vi "Die_Roller.vi"() -> ()   [LabVIEW 2020]
panel:
  out "FACE OCCURRENCES":T1
  out "Throws":dbl[](array[numeric])
  in  "Numeri Lanci":i32
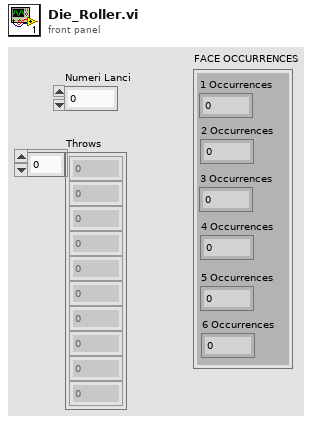
[diagram p1: front panel]
types:
  T1 = cluster{"1 Occurrences":dbl, "2 Occurrences":dbl, "3 Occurrences":dbl, "4 Occurrences":dbl, "5 Occurrences":dbl, "6 Occurrences":dbl}
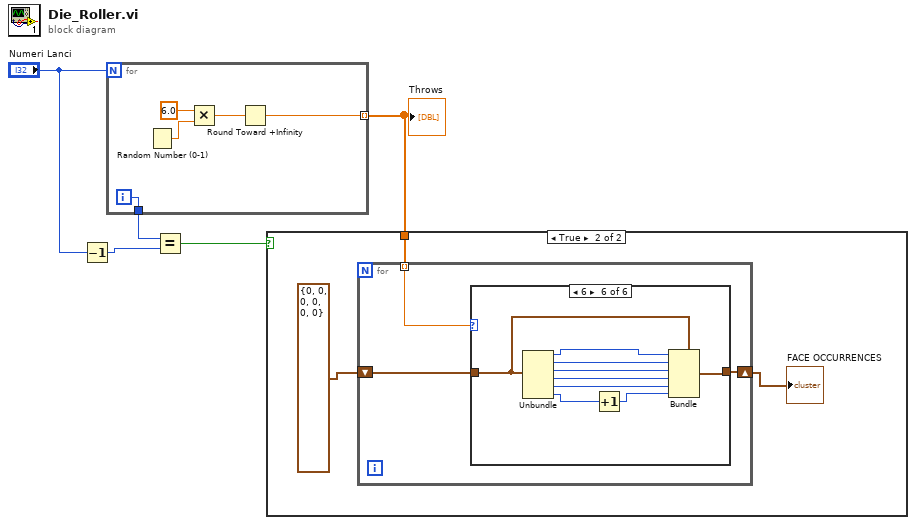
[diagram p0: block diagram]
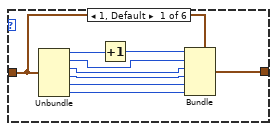
[diagram p3: hidden frame]
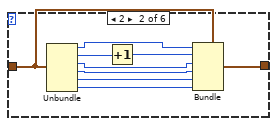
[diagram p4: hidden frame]
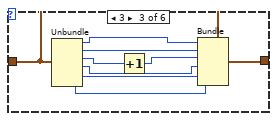
[diagram p5: hidden frame]
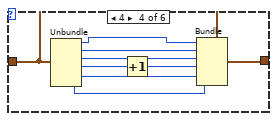
[diagram p6: hidden frame]
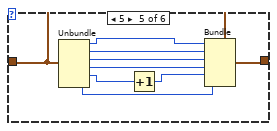
[diagram p7: hidden frame]
diagram:
  n1 = Decrement(x="Numeri Lanci") -> (x-1=w4:i32)
  n2 = for {
    N: "Numeri Lanci" -> [_]
    tunnel: [w7] -> w1 mode=indexing
    tunnel: [w6] -> w3
    i -> [w6]
    n3 = Random Number (0-1)() -> (number: 0 to 1=w10:dbl)
    n4 = Multiply(x=6.0, y=w10) -> (x*y=w8:dbl)
    n5 = Round Toward +Infinity(x=w8) -> (ceil(x): smallest int >= x=w7:dbl)
  }
  "Throws" <- w1
  n6 = Equal?(x=w3, y=w4) -> (x = y?=w2:bool)
  n7 = case shown="True" w2 {
    tunnel: w1 -> [_ w13]
    frame False {
    }
    frame True {
      n8 = for {
        tunnel: w13 -> [w16] mode=indexing
        shift-right: [w14] -> w11
        shift-left: cluster{i32, i32, i32, i32, i32, i32} {0, 0, 0, 0, 0, 0} -> [w15]
        n9 = case shown="6" w16 {
          tunnel: w15 -> [w25 w30 w39 w48 w57 w66]
          tunnel: [w17 w29 w38 w47 w56 w65] -> w14
          frame 1, Default {
            n10 = Unbundle(w25) -> (w24:i32, w22:i32, w21:i32, w20:i32, w19:i32, w18:i32)
            n11 = Increment(x=w24) -> (x+1=w23:i32)
            n12 = Bundle(cluster=w25, w23, w22, w21, w20, w19, w18) -> (w17:cluster{i32, i32, i32, i32, i32, i32})
          }
          frame 2 {
            n13 = Unbundle(w30) -> (w28:i32, w27:i32, w34:i32, w33:i32, w32:i32, w31:i32)
            n14 = Increment(x=w27) -> (x+1=w26:i32)
            n15 = Bundle(cluster=w30, w28, w26, w34, w33, w32, w31) -> (w29:cluster{i32, i32, i32, i32, i32, i32})
          }
          frame 3 {
            n16 = Unbundle(w39) -> (w40:i32, w37:i32, w36:i32, w43:i32, w42:i32, w41:i32)
            n17 = Increment(x=w36) -> (x+1=w35:i32)
            n18 = Bundle(cluster=w39, w40, w37, w35, w43, w42, w41) -> (w38:cluster{i32, i32, i32, i32, i32, i32})
          }
          frame 4 {
            n19 = Unbundle(w48) -> (w50:i32, w49:i32, w46:i32, w45:i32, w52:i32, w51:i32)
            n20 = Increment(x=w45) -> (x+1=w44:i32)
            n21 = Bundle(cluster=w48, w50, w49, w46, w44, w52, w51) -> (w47:cluster{i32, i32, i32, i32, i32, i32})
          }
          frame 5 {
            n22 = Unbundle(w57) -> (w60:i32, w59:i32, w58:i32, w55:i32, w54:i32, w61:i32)
            n23 = Increment(x=w54) -> (x+1=w53:i32)
            n24 = Bundle(cluster=w57, w60, w59, w58, w55, w53, w61) -> (w56:cluster{i32, i32, i32, i32, i32, i32})
          }
          frame 6 {
            n25 = Unbundle(w66) -> (w70:i32, w69:i32, w68:i32, w67:i32, w64:i32, w63:i32)
            n26 = Increment(x=w63) -> (x+1=w62:i32)
            n27 = Bundle(cluster=w66, w70, w69, w68, w67, w64, w62) -> (w65:cluster{i32, i32, i32, i32, i32, i32})
          }
        }
      }
      "FACE OCCURRENCES" <- w11
    }
  }
